vi "Get Number of Slots.vi"(8 "error in":errorcluster, 11 "chassis ref in":T1 format="%.0x") -> (0 "error out":errorcluster, 2 "number of slots":i32, 3 "chassis ref out":T1 format="%.0x")   [LabVIEW 2020, in "Scan Engine Scripting.lvlib"]
doc: "Returns the <B>number of slots</B> from the provided chassis reference."
uses:
  Scan Engine Scripting.lvlib
  <vilib>/NI VeriStand/Custom Device API/Custom Device Item Ref.ctl
  Scan Engine Dependencies.llb/Property Strings.vi
  <vilib>/NI VeriStand/Custom Device API/Get Item Property (I32).vi
  <vilib>/NI VeriStand/Custom Device API/Custom Device API.lvlib
  Scan Engine Dependencies.llb/Scan Engine Custom Device.lvlib
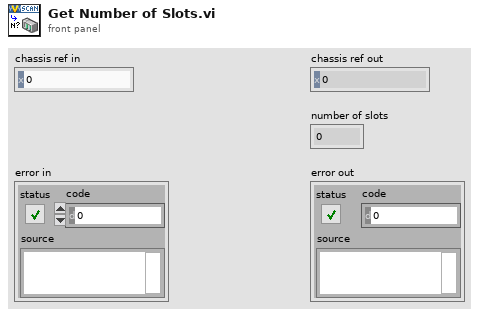
[diagram p1: front panel]
types:
  T1 = typedef "Custom Device API.lvlib/Custom Device Item Ref.ctl" = u64
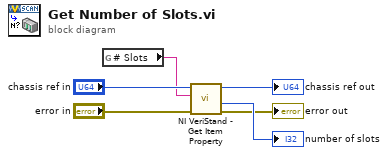
[diagram p0: block diagram]
diagram:
  n1 = global read "Property Strings.vi" "# Slots"() -> (w4:string)
  n2 = call-poly <vilib>:"NI VeriStand - Get Item Property.vi"("error in (no error)"="error in", "Property Name"=w4, "Item Ref in"="chassis ref in") -> ("error out"=→"error out":errorcluster, "Value"=→"number of slots":i32, "Item Ref out"=→"chassis ref out":T1)  [unwired: 5 in, 1 out]
